vi "Project.Open.vi"(8 "password":string, 9 "username":string, 10 "Project File Path":path, 11 "Gateway IP Address (\"\": localhost)":string) -> (0 "error out":errorcluster)   [LabVIEW 2013, in "MiscHelperVIs.lvlib"]
uses:
  MiscHelperVIs.lvlib
  NationalInstruments.VeriStand.ClientAPI
  NationalInstruments.VeriStand
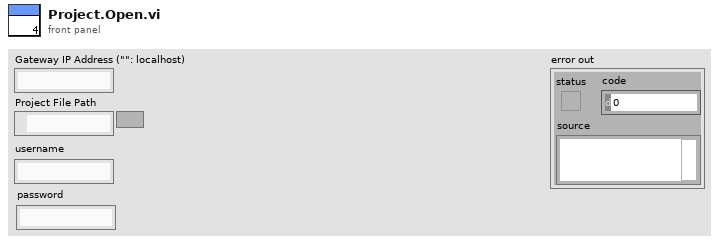
[diagram p1: front panel]
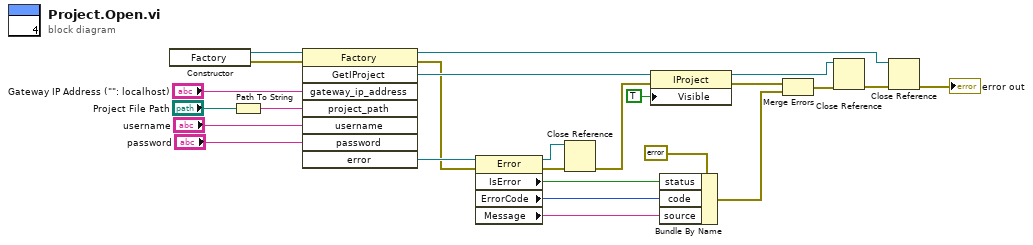
[diagram p0: block diagram]
diagram:
  n1 = constructor class="Factory"() -> (reference out=w25:refnum<k24>, error out=w17:errorcluster)  [unwired: 3 in, 1 out]
  n2 = Path To String(path="Project File Path") -> (string=w22:string)
  n3 = invoke class="Factory" method="GetIProject"(reference=w25, error in=w17, "gateway_ip_address"="Gateway IP Address (\"\": localhost)", "project_path"=w22, "username"="username", "password"="password") -> (reference out=w3:refnum<k24>, error out=w15:errorcluster, "GetIProject"=w19:refnum<k24>, "error"=w16:refnum<k24>)  [unwired: 2 in, 4 out]
  n4 = property class="Error"(reference=w16, error in=w15) -> (reference out=w8:refnum<k24>, error out=w9:errorcluster, "IsError"=w13:bool, "ErrorCode"=w12:i32, "Message"=w11:string)
  n5 = Close Reference(reference=w8, error in (no error)=w9) -> (error out=w7:errorcluster)
  n6 = property class="IProject"(reference=w19, error in=w7, "Visible"=TRUE) -> (reference out=w4:refnum<k24>, error out=w6:errorcluster)
  n7 = Bundle By Name(cluster=errorcluster {"status"=FALSE, "code"=0, "source"=""} ("error constant"), "status"=w13, "code"=w12, "source"=w11) -> (w10:errorcluster)
  n8 = Merge Errors(w6, w10) -> (w5:errorcluster)
  n9 = Close Reference(reference=w4, error in (no error)=w5) -> (error out=w2:errorcluster)
  n10 = Close Reference(reference=w3, error in (no error)=w2) -> (error out=→"error out":errorcluster)
